vi "Popup Menu Update Items.vi"(7 "Menu Items":string[](array[string]), 11 "Error In":errorcluster) -> (15 "Error Out":errorcluster)   [LabVIEW 2020]
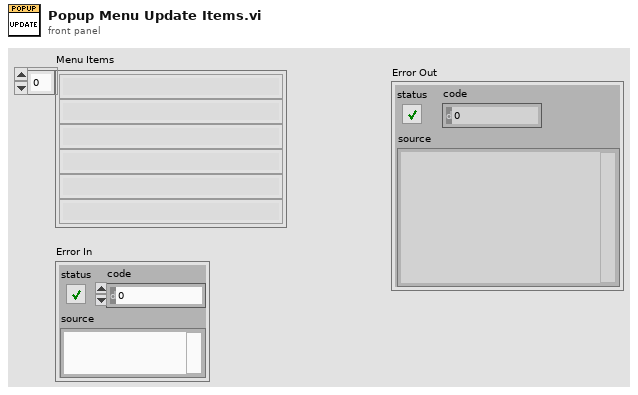
[diagram p1: front panel]
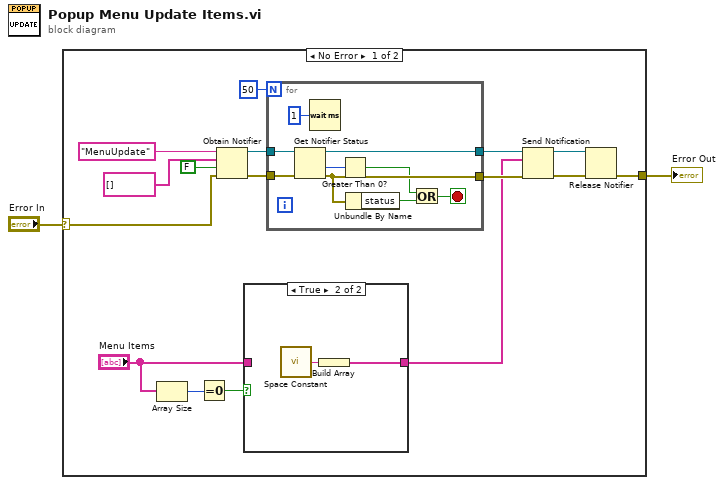
[diagram p0: block diagram]
diagram:
  n1 = case shown="No Error" "Error In" {
    selector: "Error In" -> [w7 w31]
    tunnel: [w8 w31] -> w2
    frame No Error {
      n2 = Array Size(array="Menu Items") -> (size(s)=w6:i32)
      n3 = Equal To 0?(x=w6) -> (x = 0?=w5:bool)
      n4 = Obtain Notifier(name (unnamed)="MenuUpdate", notification data type=string[] [], create if not found? (T)=FALSE, error in (no error)=w7) -> (notifier out=w15:refnum<notifier>, error out=w14:errorcluster)  [unwired: 1 out]
      n5 = case shown="True" w5 {
        tunnel: "Menu Items" -> [w19 _]
        tunnel: [w19 w20] -> w3
        frame False {
        }
        frame True {
          n6 = call <vilib>:"Space Constant.vi"() -> ("String"=w21:string)
          n7 = Build Array(w21) -> (w20:string[])
        }
      }
      n8 = for {
        N: 50 -> [_]
        tunnel: w15 -> [w30]
        tunnel: w14 -> [w29]
        tunnel: [w27] -> w12
        tunnel: [w25] -> w11
        stop <- w24 stop-if-true
        n9 = Get Notifier Status(notifier=w30, error in (no error)=w29) -> (notifier out=w27:refnum<notifier>, # waiting=w28:i32, error out=w25:errorcluster)  [unwired: 2 out]
        n10 = Wait (ms)(milliseconds to wait=u32 1) -> ()  [unwired: 1 out]
        n11 = Greater Than 0?(x=w28) -> (x > 0?=w23:bool)
        n12 = Unbundle By Name(w25) -> ("status"=w22:bool)
        n13 = Or(x=w23, y=w22) -> (x .or. y?=w24:bool)
      }
      n14 = Send Notification(notification=w3, notifier=w12, error in (no error)=w11) -> (notifier out=w10:refnum<notifier>, error out=w9:errorcluster)
      n15 = Release Notifier(notifier=w10, error in (no error)=w9) -> (error out=w8:errorcluster)  [unwired: 1 in, 2 out]
    }
    frame Error {
    }
  }
  "Error Out" <- w2
